vi "GoToHeight.vi"(6 "Synchronization":enum16{"Start", "Wait"}(ring), 7 "Description":string, 8 "Command Info In":T1, 9 "Setpoint":dbl) -> (0 "Command Info Out":T1)   [LabVIEW 2017]
doc: "This template has a parameter to control whether it waits for the command to complete or not. This is useful for operations that have a timed duration or a sensor-based duration. \n\nBe sure to right-click and select New from Template and save with a new command name."
uses:
  <vilib>/Rock Robotics/WPI/Framework/Command Status Info.ctl
  <vilib>/Rock Robotics/WPI/Framework/Completion Status.ctl
  <vilib>/Rock Robotics/WPI/Framework/Completion Notifier.ctl
  Implementation/Elevator Setpoints.ctl
  Implementation/Elevator Operations.ctl
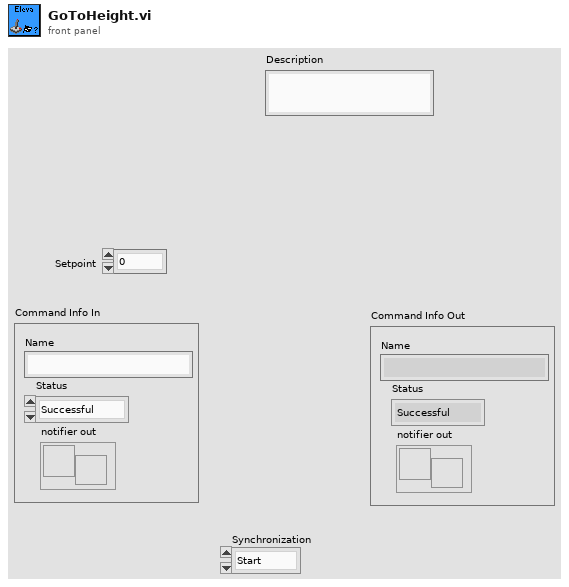
[diagram p1: front panel]
types:
  T1 = typedef "Command Status Info.ctl" = cluster{"Name":string, "Status":T2, "notifier out":T3}
  T2 = typedef "Completion Status.ctl" = enum16{"Successful", "Aborted", "Incomplete"}
  T3 = typedef "Completion Notifier.ctl" = refnum<notifier>
  T4 = typedef "Elevator Operations.ctl" = enum16{"Reserve", "Read Current", "Immediate", "GoToHeight", "StayAtHeight", "LiftForTime"}
  T5 = typedef "Elevator Setpoints.ctl" = cluster{"Operation":T4, "Setpoint":dbl, "Duration":dbl, "Button":bool}
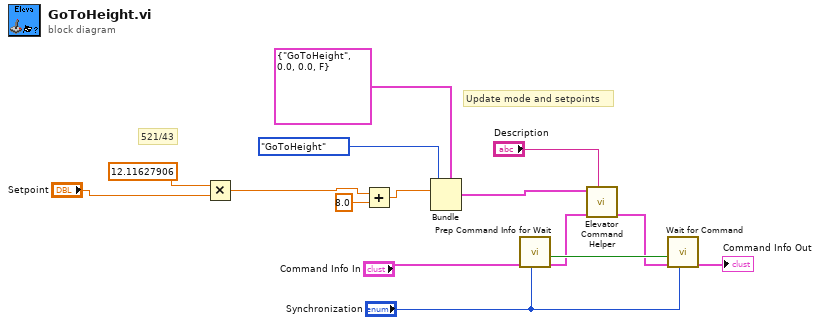
[diagram p0: block diagram]
diagram:
  # "521/43"
  # "Update mode and setpoints"
  n1 = Multiply(x=12.11627906, y="Setpoint") -> (x*y=w2:dbl)
  n2 = Add(x=w2, y=8.0) -> (x+y=w1:dbl)
  n3 = Bundle(cluster=T5 {"Operation"=enum."GoToHeight", "Setpoint"=0.0, "Duration"=0.0, "Button"=FALSE} ("SubSystem Data"), "Operation"=Elevator_Operations."GoToHeight", "Setpoint"=w1) -> (w8:T5)  [unwired: 2 in]
  n4 = call <vilib>:"Prep Command Info for Wait.vi"("Synchronication"="Synchronization", "Command Info"="Command Info In") -> ("Command Info"=w12:T1, "Allocated"=w13:bool)  [unwired: 8 in]
  n5 = call "Elevator Command Helper.vi"("Description"="Description", "Command Info In"=w12, "SubSystem Data"=w8) -> ("Command Info Out"=w9:T1)  [unwired: 6 in, 2 out]
  n6 = call <vilib>:"Wait for Command.vi"("Synchronication"="Synchronization", "Command Info in"=w9, "Allocated"=w13) -> ("Command Info out"=→"Command Info Out":T1)  [unwired: 8 in]
